vi "Check if Subpanel Tag.vi"(8 "error in":errorcluster, 10 "subpanel tag":string, 11 "state in":T1) -> (0 "error out":errorcluster, 1 "owning VI name":string, 2 "found?":bool, 3 "state out":T1, 4 "subpanel UID":i32)   [LabVIEW 2010, in "NI_SE_Config Front Panel Layout.lvlib"]
uses:
  NI_SE_Config Front Panel Layout.lvlib
  State.ctl
  VI Info.ctl
  VI Panel Layout/VI Panel Layout.lvclass
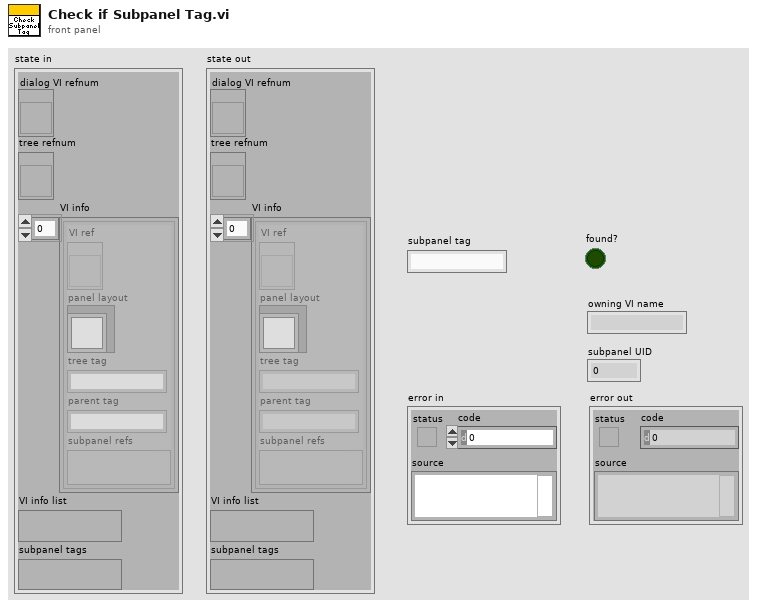
[diagram p1: front panel]
types:
  T1 = typedef "NI_SE_Config Front Panel Layout.lvlib/State.ctl" = cluster{"dialog VI refnum":refnum<vi>, "tree refnum":refnum<vi>, "VI info":T2[], "VI info list":variant, "subpanel tags":variant}
  T2 = typedef "NI_SE_Config Front Panel Layout.lvlib/VI Info.ctl" = cluster{"VI ref":refnum<vi>, "panel layout":refnum<class "VI Panel Layout.lvclass">, "tree tag":string, "parent tag":string, "subpanel refs":variant}
  T3 = cluster{"subpanel UID":i32, "owning VI name":string}
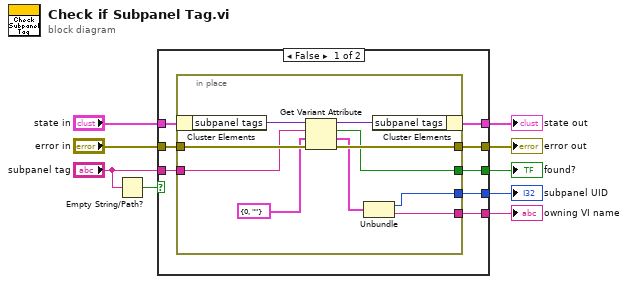
[diagram p0: block diagram]
diagram:
  n1 = Empty String/Path?(string/path="subpanel tag") -> (empty?=w1:bool)
  n2 = case shown="False" w1 {
    tunnel: "state in" -> [w17 w29]
    tunnel: "subpanel tag" -> [w16 _]
    tunnel: "error in" -> [w15 w28]
    tunnel: [w14 w29] -> w7
    tunnel: [w13 w28] -> w6
    tunnel: [w12 _] -> w5
    tunnel: [w11 _] -> w4
    tunnel: [w10 _] -> w3
    frame False {
      n3 = in-place {
        in-place-border: w16 -> [w23]
        in-place-border: w15 -> [w25]
        in-place-border: [w24] -> w13
        in-place-border: [w22] -> w12
        in-place-border: [w20] -> w11
        in-place-border: [w19] -> w10
        n4 = in-place-cluster #1(w17) -> ("subpanel tags"=w27:variant)
        n5 = Get Variant Attribute(Variant=w27, name=w23, default value (empty Variant)=T3 {"subpanel UID"=0, "owning VI name"=""} ("output cluster"), error in=w25) -> (duplicate Variant=w26:variant, found=w22:bool, value=w21:T3, error out=w24:errorcluster)
        n6 = Unbundle(w21) -> ("subpanel UID"=w19:i32, "owning VI name"=w20:string)
        n7 = in-place-cluster #1("subpanel tags"=w26) -> (w14:T1)
      }
    }
    frame True {
    }
  }
  "state out" <- w7
  "error out" <- w6
  "found?" <- w5
  "owning VI name" <- w4
  "subpanel UID" <- w3
